vi "Options Dialog.vi"(11 "State In":T1) -> (3 "State Out":T1)   [LabVIEW 2018, in "RetryNode.xnode"]
uses:
  RetryNode.xnode
  State.ctl
  <vilib>/Utility/miscctls.llb/LVRectTypeDef.ctl
  Options.ctl
panel:
  in  "Max retries":i32=-1
  in  "Enable Retry":bool=TRUE
  in  "Retry VI Path":path
  in  "OK":bool
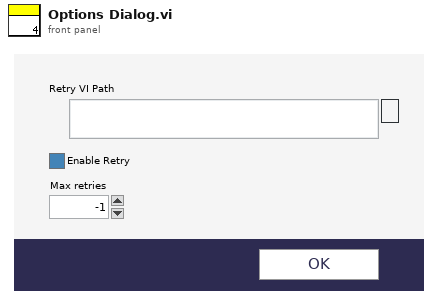
[diagram p1: front panel]
types:
  T1 = typedef "RetryNode.xnode/State.ctl" = cluster{"RetryVI path":path, "TerminalState":cluster{"ID":i32, "Type":variant, "Name":string, "Input?":bool, "Term Limits":T2, "Wire Rule":enum16{"Invalid Wire Rule", "Required", "Recommended", "Optional", "Dynamic Dispatch"}, "Wired ?":bool}[], "Retry Options":T3}
  T2 = typedef "LVRectTypeDef.ctl" = cluster{"Left":i16, "Top":i16, "Right":i16, "Bottom":i16}
  T3 = typedef "RetryNode.xnode/Options.ctl" = cluster{"Enable":bool, "Max Retries":i32}
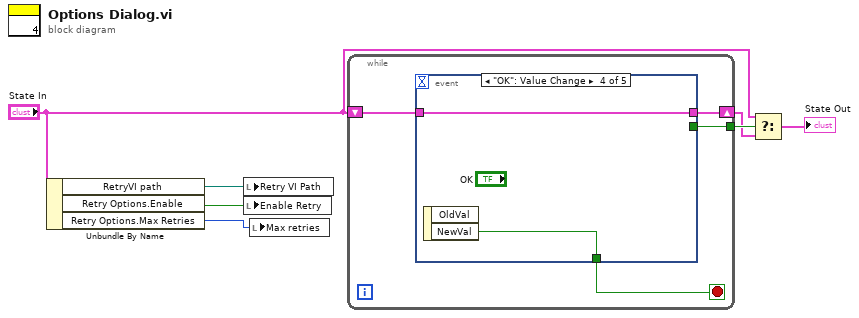
[diagram p0: block diagram]
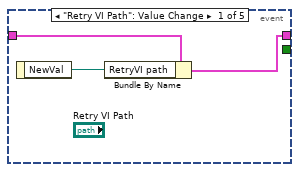
[diagram p2: hidden frame]
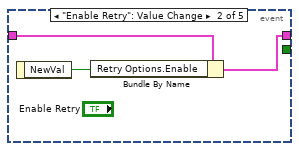
[diagram p3: hidden frame]
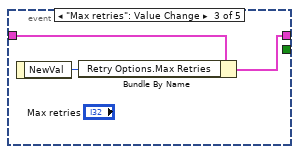
[diagram p4: hidden frame]
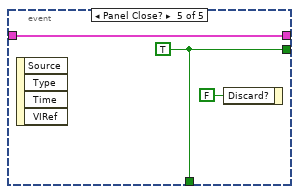
[diagram p5: hidden frame]
diagram:
  n1 = Unbundle By Name("State In") -> ("RetryVI path"=w3:path, "Retry Options.Enable"=w2:bool, "Retry Options.Max Retries"=w1:i32)
  n2 = local write "Retry VI Path"(w3) -> ()
  n3 = local write "Enable Retry"(w2) -> ()
  n4 = local write "Max retries"(w1) -> ()
  n5 = while {
    tunnel: [w9] -> w7
    shift-right: [w8] -> w6
    shift-left: "State In" -> [w10]
    stop <- w11 stop-if-true
    n6 = event shown="[3] \"OK\": Value Change" {
      selector: _ -> [_ _ _ _ _]
      dyn-events: _ -> [_ _ _ _ _]
      timeout: _ -> [_ _ _ _ _]
      tunnel: [_ _ _ w22 w24] -> w11
      tunnel: w10 -> [w14 w17 w20 w21 w23]
      tunnel: [_ _ _ _ w24] -> w9
      tunnel: [w12 w15 w18 w21 w23] -> w8
      event "Retry VI Path": Value Change {
        n7 = event-data() -> ("NewVal"=w13:path)  [unwired: 1 in]
        n8 = Bundle By Name(cluster=w14, "RetryVI path"=w13) -> (w12:T1)
      }
      event "Enable Retry": Value Change {
        n9 = event-data() -> ("NewVal"=w16:bool)  [unwired: 1 in]
        n10 = Bundle By Name(cluster=w17, "Retry Options.Enable"=w16) -> (w15:T1)
      }
      event "Max retries": Value Change {
        n11 = event-data() -> ("NewVal"=w19:i32)  [unwired: 1 in]
        n12 = Bundle By Name(cluster=w20, "Retry Options.Max Retries"=w19) -> (w18:T1)
      }
      event "OK": Value Change {
        n13 = event-data() -> ("NewVal"=w22:bool)  [unwired: 1 in, 1 out]
      }
      event Panel Close? {
        w24 = TRUE ("Discard?")
        n14 = event-data() -> ()  [unwired: 1 in, 4 out]
        n15 = event-data("Discard?"=FALSE) -> ()  [unwired: 1 in, 1 out]
      }
    }
  }
  n16 = Select(t="State In", s=w7, f=w6) -> (s? t:f=→"State Out":T1)
